vi "Get Type.vi"(8 "error in (no error)":errorcluster, 11 "Library Instr in":refnum<class "Library Instr.lvclass">) -> (0 "error out":errorcluster, 2 "Type":string, 3 "Library Instr out":refnum<class "Library Instr.lvclass">)   [LabVIEW 2015, in "Item Actor.lvlib" / "Library Instr.lvclass"]
uses:
  Library Instr.lvclass
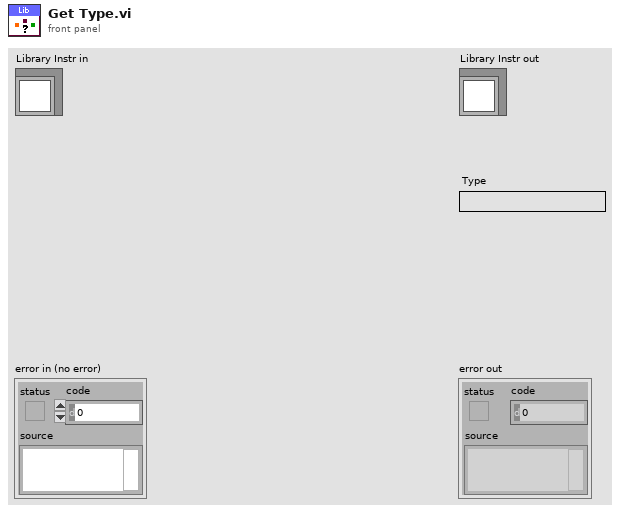
[diagram p1: front panel]
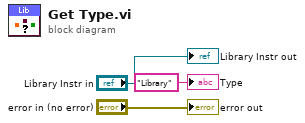
[diagram p0: block diagram]
diagram:
  "error out" <- "error in (no error)"
  "Library Instr out" <- "Library Instr in"
  "Type" <- "Library" ("Type")
